vi "test_dragon_file--read_package_states_toml.vi"(8 "error in (no error)":errorcluster) -> (0 "error out":errorcluster)   [LabVIEW 2020]
uses:
  57e33671-8226-461a-9661-efe5b126b970.vi
  e7350a7c-a60d-45e2-883c-19031d0482ee.vi
  8e2fd1fc-adf1-4514-8afa-9b03396949d3.vi
  4d723e19-c997-45c0-974f-972ac2757a32.vi
  e5cc773a-9f3c-4ead-839d-2efea4be6060.vi
  57e33671-8226-461a-9661-efe5b126b970.vi/05157253-4ade-4b75-9902-c642c5dd4762.vi
  57e33671-8226-461a-9661-efe5b126b970.vi/543db544-a529-4041-9332-0fe0cbee0c9f.vi
  57e33671-8226-461a-9661-efe5b126b970.vi/3109fa46-d519-4eec-8db6-6c1d337e5c6d.vi
  e7350a7c-a60d-45e2-883c-19031d0482ee.vi/05157253-4ade-4b75-9902-c642c5dd4762.vi
  e7350a7c-a60d-45e2-883c-19031d0482ee.vi/543db544-a529-4041-9332-0fe0cbee0c9f.vi
  e7350a7c-a60d-45e2-883c-19031d0482ee.vi/3109fa46-d519-4eec-8db6-6c1d337e5c6d.vi
  8e2fd1fc-adf1-4514-8afa-9b03396949d3.vi/05157253-4ade-4b75-9902-c642c5dd4762.vi
  8e2fd1fc-adf1-4514-8afa-9b03396949d3.vi/543db544-a529-4041-9332-0fe0cbee0c9f.vi
  8e2fd1fc-adf1-4514-8afa-9b03396949d3.vi/3109fa46-d519-4eec-8db6-6c1d337e5c6d.vi
  4d723e19-c997-45c0-974f-972ac2757a32.vi/05157253-4ade-4b75-9902-c642c5dd4762.vi
  4d723e19-c997-45c0-974f-972ac2757a32.vi/543db544-a529-4041-9332-0fe0cbee0c9f.vi
  4d723e19-c997-45c0-974f-972ac2757a32.vi/3109fa46-d519-4eec-8db6-6c1d337e5c6d.vi
  e5cc773a-9f3c-4ead-839d-2efea4be6060.vi/05157253-4ade-4b75-9902-c642c5dd4762.vi
  e5cc773a-9f3c-4ead-839d-2efea4be6060.vi/543db544-a529-4041-9332-0fe0cbee0c9f.vi
  e5cc773a-9f3c-4ead-839d-2efea4be6060.vi/3109fa46-d519-4eec-8db6-6c1d337e5c6d.vi
  toml/read_subtable_item.vi
  Item/get_item_type.vi
  Item/to_value.vi
  Value/get_value_type.vi
  Value/get_value_for_string.vi
  Value/get_value_for_integer.vi
  Value/get_value_for_boolean.vi
  toml/toml.lvclass
  <vilib>/addons/_JKI Toolkits/Caraya/classes/Assert/Assert.lvclass
  <vilib>/addons/_JKI Toolkits/Caraya/classes/Test/Test.lvclass
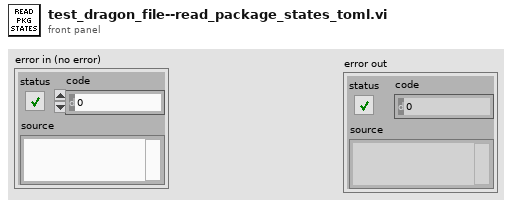
[diagram p1: front panel]
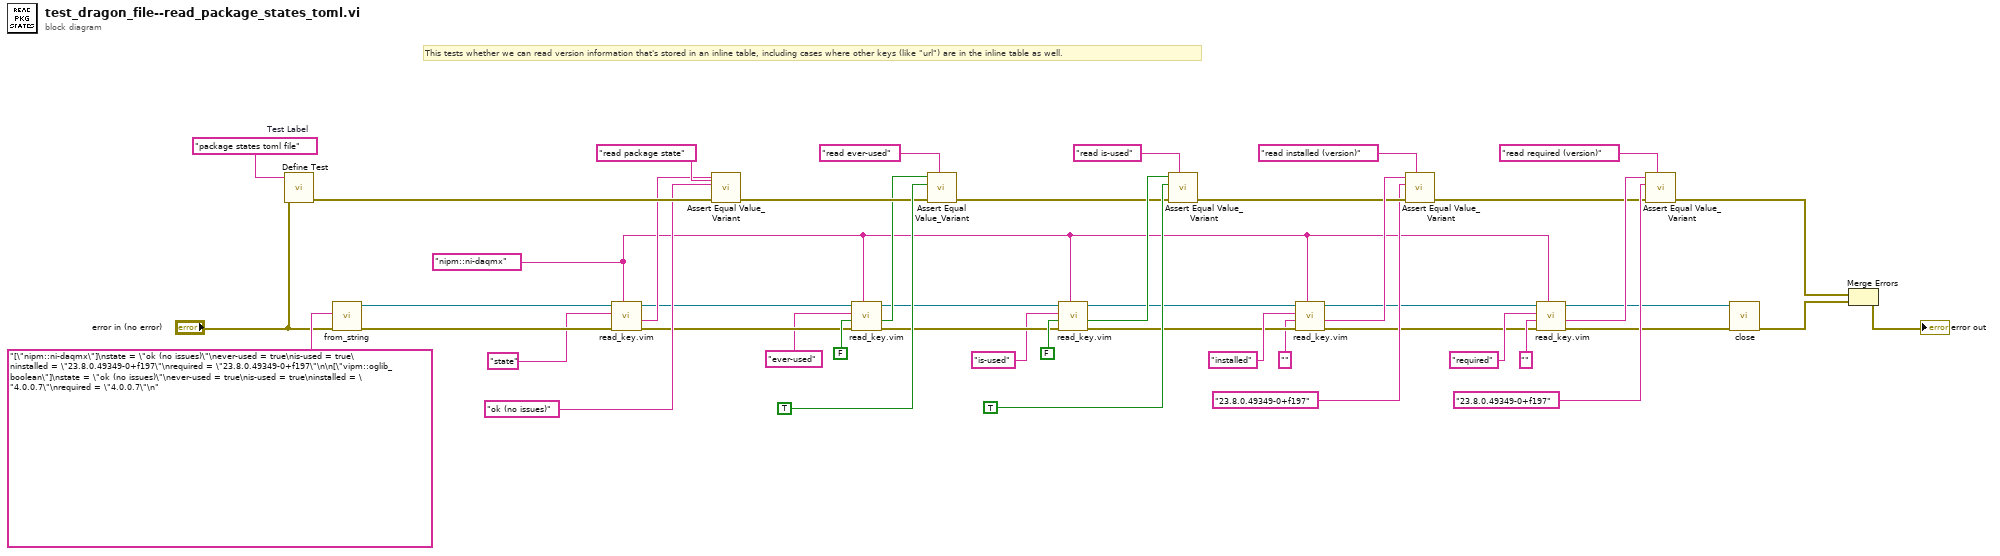
[diagram p0: block diagram]
diagram:
  w4 = "nipm::ni-daqmx" ("table_name")
  w44 = "package states toml file"  # Test Label
  # "This tests whether we can read version information that's stored in an inline table, including cases where other keys (like \"url\") are in the inline table as well."
  n1 = call <vilib>:"Define Test.vi"("error in (no error)"="error in (no error)", "Label (VI Title)"=w44) -> ("error out"=w45:errorcluster)  [unwired: 8 in, 1 out]
  n2 = call "from_string.vi"("error in (no error)"="error in (no error)", "toml"="[\"nipm::ni-daqmx\"]\nstate = \"ok (no issues)\"\never-used = true\nis-used = true\ninstalled = \"23.8.0.49349-0+f197\"\nrequired = \"23.8.0.49349-0+f197\"\n\n[\"vipm::oglib_boolean\"]\nstate = \"ok (no issues)\"\never-used = true\nis-used = true\ninstalled = \"4.0.0.7\"\nrequired = \"4.0.0.7\"\n" ("toml_string in")) -> ("error out"=w42:errorcluster, "toml out"=w43:refnum<class "toml.lvclass">)  [unwired: 8 in]
  n3 = call "read_key.vim"("table"=w4, "error in (no error)"=w42, "key"="state" ("table_name"), "toml in"=w43) -> ("error out"=w32:errorcluster, "value"=w39:string, "toml out"=w33:refnum<class "toml.lvclass">)  [unwired: 4 in, 1 out]
  n4 = call <vilib>:"Assert Equal Value_Variant.vi"("Label"="read package state", "error in (no error)"=w45, "Y"="ok (no issues)" ("table_name"), "X"=w39) -> ("error out"=w35:errorcluster)  [unwired: 6 in, 1 out]
  n5 = call "read_key.vim"("table"=w4, "error in (no error)"=w32, "default (\"\")"=FALSE, "key"="ever-used" ("table_name"), "toml in"=w33) -> ("error out"=w28:errorcluster, "value"=w31:bool, "toml out"=w29:refnum<class "toml.lvclass">)  [unwired: 3 in, 1 out]
  n6 = call <vilib>:"Assert Equal Value_Variant.vi"("Label"="read ever-used", "error in (no error)"=w35, "Y"=TRUE, "X"=w31) -> ("error out"=w24:errorcluster)  [unwired: 6 in, 1 out]
  n7 = call "read_key.vim"("table"=w4, "error in (no error)"=w28, "default (\"\")"=FALSE, "key"="is-used" ("table_name"), "toml in"=w29) -> ("error out"=w16:errorcluster, "value"=w26:bool, "toml out"=w17:refnum<class "toml.lvclass">)  [unwired: 3 in, 1 out]
  n8 = call <vilib>:"Assert Equal Value_Variant.vi"("Label"="read is-used", "error in (no error)"=w24, "Y"=TRUE, "X"=w26) -> ("error out"=w15:errorcluster)  [unwired: 6 in, 1 out]
  n9 = call "read_key.vim"("table"=w4, "error in (no error)"=w16, "default (\"\")"="" ("table_name"), "key"="installed" ("table_name"), "toml in"=w17) -> ("error out"=w5:errorcluster, "value"=w19:string, "toml out"=w6:refnum<class "toml.lvclass">)  [unwired: 3 in, 1 out]
  n10 = call <vilib>:"Assert Equal Value_Variant.vi"("Label"="read installed (version)", "error in (no error)"=w15, "Y"="23.8.0.49349-0+f197" ("table_name"), "X"=w19) -> ("error out"=w7:errorcluster)  [unwired: 6 in, 1 out]
  n11 = call "read_key.vim"("table"=w4, "error in (no error)"=w5, "default (\"\")"="" ("table_name"), "key"="required" ("table_name"), "toml in"=w6) -> ("error out"=w2:errorcluster, "value"=w11:string, "toml out"=w1:refnum<class "toml.lvclass">)  [unwired: 3 in, 1 out]
  n12 = call <vilib>:"Assert Equal Value_Variant.vi"("Label"="read required (version)", "error in (no error)"=w7, "Y"="23.8.0.49349-0+f197" ("table_name"), "X"=w11) -> ("error out"=w3:errorcluster)  [unwired: 6 in, 1 out]
  n13 = call "close.vi"("error in (no error)"=w2, "toml in"=w1) -> ("error out"=w41:errorcluster)  [unwired: 9 in]
  n14 = Merge Errors(w3, w41) -> (→"error out":errorcluster)
